vi "Define Ephemeral Strategies.vi"(7 "Clear":bool, 10 "Ephemeral Strategies":map{string, refnum<class "BananaPeel.lvclass">}(c390), 11 "Banana in":refnum<class "Banana.lvclass">) -> (1 "update":bool, 3 "Banana":refnum<class "Banana.lvclass">)   [LabVIEW 2021, in "Bananas.lvlib" / "Banana.lvclass"]
uses:
  Banana.lvclass
  Banana.lvclass/Banana.ctl
  Platano/Platano.lvclass
  BananaPeel/BananaPeel.lvclass
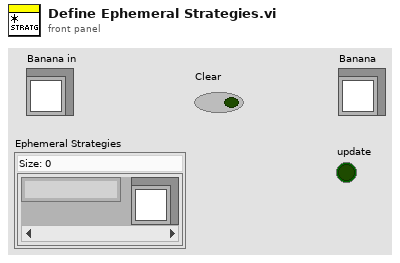
[diagram p1: front panel]
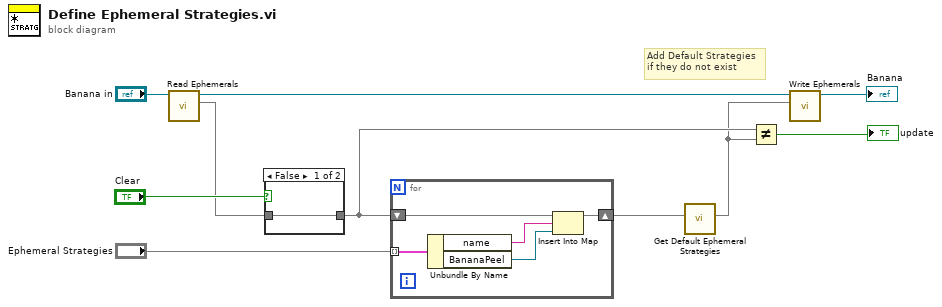
[diagram p0: block diagram]
diagram:
  # "Add Default Strategies\nif they do not exist"
  n1 = call "Read Ephemerals.vi"("Banana in"="Banana in") -> ("Ephemerals"=w5:map{string, refnum<class "BananaPeel.lvclass">}, "Banana out"=w3:refnum<class "Banana.lvclass">)  [unwired: 8 in, 1 out]
  n2 = case shown="False" "Clear" {
    tunnel: [w11 _] -> w6
    tunnel: w5 -> [w11 _]
    frame False {
    }
    frame True {
    }
  }
  n3 = for {
    shift-right: [w14] -> w9
    shift-left: w6 -> [w15]
    tunnel: "Ephemeral Strategies" -> [w16] mode=indexing
    n4 = Unbundle By Name(w16) -> ("name"=w13:string, "BananaPeel"=w12:refnum<class "BananaPeel.lvclass">)
    n5 = Insert Into Map(map in=w15, key=w13, value=w12) -> (map out=w14:map{string, refnum<class "BananaPeel.lvclass">})  [unwired: 2 out]
  }
  n6 = call "Get Default Ephemeral Strategies.vi"("Ephemeral Strategies in"=w9) -> ("Ephemeral Strategies"=w2:map{string, refnum<class "BananaPeel.lvclass">})  [unwired: 10 in]
  n7 = Not Equal?(x=w6, y=w2) -> (x != y?=→"update":bool)
  n8 = call "Write Ephemerals.vi"("Ephemerals"=w2, "Banana in"=w3) -> ("Banana out"=→"Banana":refnum<class "Banana.lvclass">)  [unwired: 8 in, 1 out]
